vi "read.vi"(7 "timeout (ms)":i32, 8 "error in (no error)":errorcluster, 9 "number of channels":i32, 10 "block size":i32, 11 "FPGAWrapperDL090211Galvo in":refnum<class "FPGAWrapperDL090211Galvo.lvclass">) -> (0 "error out":errorcluster, 1 "channels raw data block":T1, 2 "FIFO full?":bool, 3 "FPGAWrapperDL090211Galvo out":refnum<class "FPGAWrapperDL090211Galvo.lvclass">, 4 "timed out?":bool)   [LabVIEW 2010, in "FPGAWrapperDL090211Galvo.lvclass"]
uses:
  FPGAWrapperDL090211Galvo.lvclass
  common/arrays/pixel_raw_data_array.ctl
  class_data.vi
  Program Files (x86)/National Instruments/LabVIEW 2010/resource/objmgr/ni.dex.rc
panel:
  out "s? t:f":dbl[][](array[numeric])
  in  "clamp?":bool
  out "available elements for reading":i32
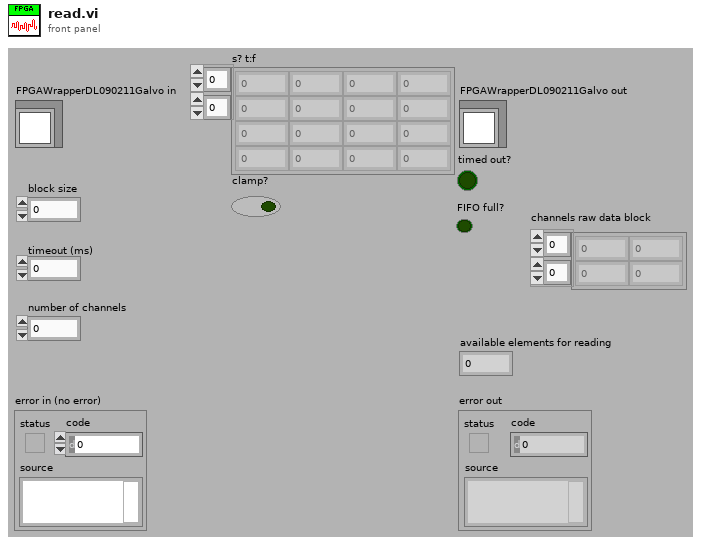
[diagram p1: front panel]
types:
  T1 = typedef "pixel_raw_data_array.ctl" = dbl[][]
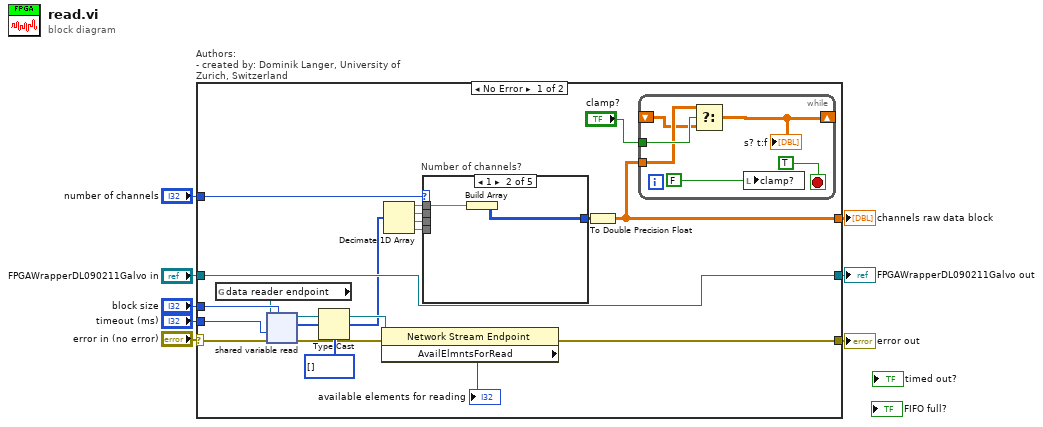
[diagram p0: block diagram]
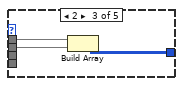
[diagram p3: hidden frame]
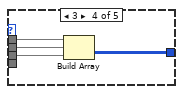
[diagram p4: hidden frame]
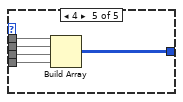
[diagram p5: hidden frame]
diagram:
  n1 = case "Authors: \n- created by: Dominik Langer, University of Zurich, Switzerland" shown="No Error" "error in (no error)" {
    selector: "error in (no error)" -> [w24 w49]
    tunnel: "FPGAWrapperDL090211Galvo in" -> [w22 w50]
    tunnel: "timeout (ms)" -> [w23 _]
    tunnel: "number of channels" -> [w28 _]
    tunnel: "block size" -> [w26 _]
    tunnel: [w18 w49] -> w3
    tunnel: [w22 w50] -> w2
    tunnel: [w10 _] -> w1
    frame No Error {
      n2 = global read "class_data.vi" "data reader endpoint"() -> (w21:refnum<k21>)
      n3 = shared-variable-read(w21, w24, w23, w26) -> (w20:refnum<k21>, w19:errorcluster, w25:u64[])  [unwired: 1 out]
      n4 = Type Cast(type=u16[] [], x=w25) -> (*(type *) &x=w16:u16[])
      n5 = property class="Network Stream Endpoint"(reference=w20, error in=w19) -> (error out=w18:errorcluster, "AvailElmntsForRead"=→"available elements for reading":i32)  [unwired: 1 out]
      n6 = Decimate 1D Array(w16) -> (w15:u16[], w14:u16[], w13:u16[], w12:u16[])
      n7 = case "Number of channels?" shown="1" w28 {
        tunnel: w15 -> [_ w35 w39 w43 w48]
        tunnel: w14 -> [_ _ w38 w42 w47]
        tunnel: w13 -> [_ _ _ w41 w46]
        tunnel: w12 -> [_ _ _ _ w45]
        tunnel: [_ w36 w37 w40 w44] -> w11
        frame 0, Default {
        }
        frame 1 {
          n8 = Build Array(w35) -> (w36:u16[][])
        }
        frame 2 {
          n9 = Build Array(w39, w38) -> (w37:u16[][])
        }
        frame 3 {
          n10 = Build Array(w43, w42, w41) -> (w40:u16[][])
        }
        frame 4 {
          n11 = Build Array(w48, w47, w46, w45) -> (w44:u16[][])
        }
      }
      n12 = To Double Precision Float(number=w11) -> (double precision float=w10:dbl[][])
      n13 = while {
        shift-right: [w29] -> _
        shift-left: _ -> [w30]
        tunnel: w10 -> [w31]
        tunnel: "clamp?" -> [w34]
        stop <- TRUE stop-if-true
        n14 = Select(t=w31, s=w34, f=w30) -> (s? t:f=w29:dbl[][])
        "s? t:f" <- w29
        n15 = local write "clamp?"(FALSE ("clamp?")) -> ()
      }
    }
    frame Error {
    }
  }
  "error out" <- w3
  "FPGAWrapperDL090211Galvo out" <- w2
  "channels raw data block" <- w1
